vi "Read Display mode.vi"(8 "error in (no error)":errorcluster, 11 "U32 D Element in":refnum<class "U32 D Element.lvclass">) -> (0 "error out":errorcluster, 2 "Display mode":T1, 3 "U32 D Element out":refnum<class "U32 D Element.lvclass">)   [LabVIEW 2018, in "D Datagrid Library.lvlib" / "U32 D Element.lvclass"]
uses:
  U32 D Element.lvclass
  Display mode.ctl
  U32 D Element.lvclass/U32 D Element.ctl
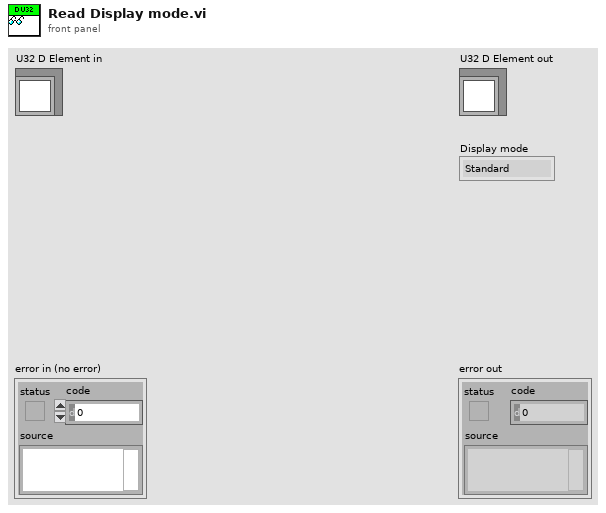
[diagram p1: front panel]
types:
  T1 = typedef "D Datagrid Library.lvlib/U32 D Element.lvclass/Display mode.ctl" = enum16{"Standard", "Hex"}
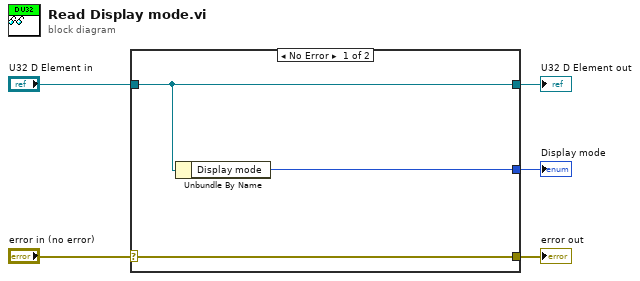
[diagram p0: block diagram]
diagram:
  n1 = case shown="No Error" "error in (no error)" {
    selector: "error in (no error)" -> [w8 w9]
    tunnel: [w8 w9] -> w4
    tunnel: [w7 w10] -> w2
    tunnel: "U32 D Element in" -> [w7 w10]
    tunnel: [w6 _] -> w1
    frame No Error {
      n2 = Unbundle By Name(w7) -> ("Display mode"=w6:T1)
    }
    frame Error {
    }
  }
  "error out" <- w4
  "U32 D Element out" <- w2
  "Display mode" <- w1
